vi "CF-common_filepath.vi"(11 "Input path":string) -> (2 "Common Path + input":path, 3 "Common Path":path)   [LabVIEW 2020, in "CF-common_features.lvlib"]
uses:
  CF-common_features.lvlib
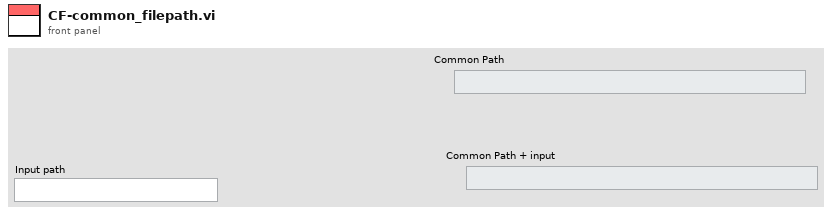
[diagram p1: front panel]
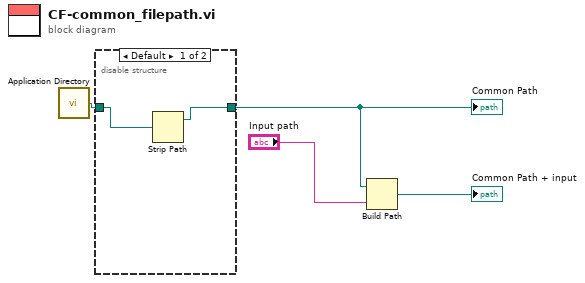
[diagram p0: block diagram]
diagram:
  n1 = call <vilib>:"Application Directory.vi"() -> ("Application Directory"=w4:path)
  n2 = disable-structure shown="Default" {
    disable-tunnel: w4 -> [w6 w7]
    disable-tunnel: [w5 w7] -> w3
    frame condition #0 (active) {
      n3 = Strip Path(path=w6) -> (stripped path=w5:path)  [unwired: 1 out]
    }
    frame condition #1 {
    }
  }
  "Common Path" <- w3
  n4 = Build Path(base path=w3, name or relative path="Input path") -> (appended path=→"Common Path + input":path)
